vi "Handle Messages.vi"(8 "error in (no error)":errorcluster, 9 "Message Data":variant, 10 "Message":string, 11 "Person In":refnum<class "Person.lvclass">) -> (0 "error out":errorcluster, 3 "Person Out":refnum<class "Person.lvclass">)   [LabVIEW 2020, in "Person.lvclass"]
uses:
  Person.lvclass
  C:/Program Files (x86)/National Instruments/LabVIEW 2020/vi.lib/Asteme/Triarc Framework/Process/Process.lvclass
  Person.lvclass/Person.ctl
  <vilib>/Asteme/Triarc Framework/Process/Process.lvclass/Process.ctl
  <vilib>/Asteme/Triarc Framework/Process/Public/Lifecycle/Get Lifecycle State.vi
  <vilib>/Utility/error.llb/Clear Errors.vi
  <vilib>/Utility/error.llb/Error Cluster From Error Code.vi
  <vilib>/Asteme/Triarc Framework/View/View.lvclass
  <vilib>/Asteme/Triarc Framework/Process/Process.lvclass
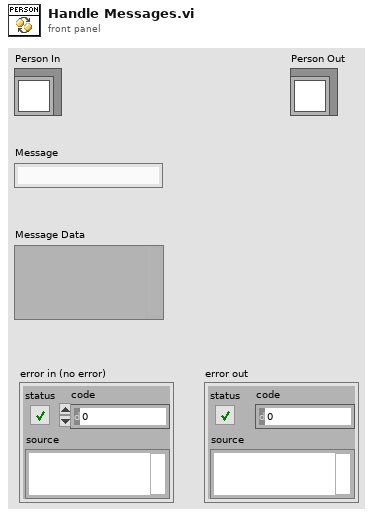
[diagram p1: front panel]
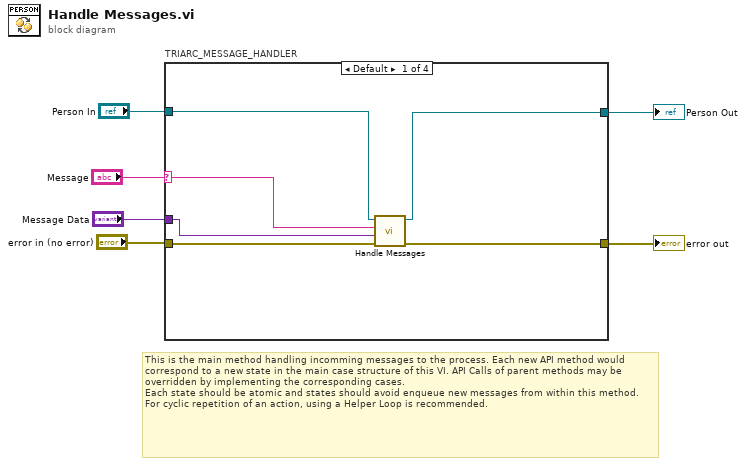
[diagram p0: block diagram]
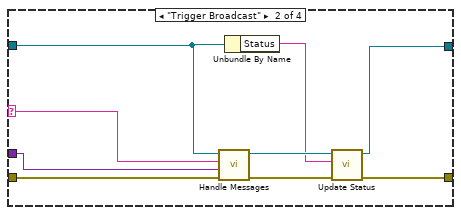
[diagram p2: hidden frame]
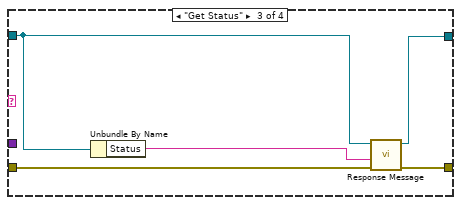
[diagram p3: hidden frame]
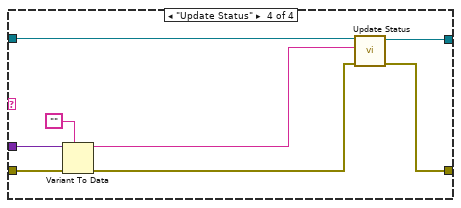
[diagram p4: hidden frame]
diagram:
  # "This is the main method handling incomming messages to the process. Each new API method would correspond to a new state in the main case structure of this VI. API Calls of parent methods may be overridden by implementing the corresponding cases.\nEach state should be atomic and states should avoid enqueue new messages from within this method. For cyclic repetition of an action, using a Helper Loop is recommended."
  n1 = case "TRIARC_MESSAGE_HANDLER" shown="Default" "Message" {
    selector: "Message" -> [w10 w20 _ _]
    tunnel: "error in (no error)" -> [w9 w19 w25 w30]
    tunnel: "Person In" -> [w12 w14 w24 w27]
    tunnel: "Message Data" -> [w11 w21 _ w33]
    tunnel: [w8 w17 w22 w28] -> w2
    tunnel: [w7 w15 w23 w29] -> w1
    frame Default {
      n2 = call-parent "Handle Messages.vi"("error in (no error)"=w9, "Message Data"=w11, "Message"=w10, "View In"=w12) -> ("error out"=w8:errorcluster, "View Out"=w7:refnum<class "Person.lvclass">)  [unwired: 6 in]
    }
    frame "Trigger Broadcast" {
      n3 = call-parent "Handle Messages.vi"("error in (no error)"=w19, "Message Data"=w21, "Message"=w20, "View In"=w14) -> ("error out"=w18:errorcluster, "View Out"=w16:refnum<class "Person.lvclass">)  [unwired: 6 in]
      n4 = Unbundle By Name(w14) -> ("Status"=w13:string)
      n5 = call "Update Status.vi"("error in (no error)"=w18, "Status"=w13, "Person In"=w16) -> ("error out"=w17:errorcluster, "Person Out"=w15:refnum<class "Person.lvclass">)  [unwired: 7 in]
    }
    frame "Get Status" {
      n6 = Unbundle By Name(w24) -> ("Status"=w26:string)
      n7 = call <vilib>:"Response Message.vi"("error in (no error)"=w25, "Response Message Data"=w26, "Process In"=w24) -> ("error out"=w22:errorcluster, "Process Out"=w23:refnum<class "Person.lvclass">)  [unwired: 7 in]
    }
    frame "Update Status" {
      n8 = Variant To Data(error in=w30, type="", Variant=w33) -> (data=w31:string, error out=w34:errorcluster)
      n9 = call "Update Status.vi"("error in (no error)"=w34, "Status"=w31, "Person In"=w27) -> ("error out"=w28:errorcluster, "Person Out"=w29:refnum<class "Person.lvclass">)  [unwired: 7 in]
    }
  }
  "error out" <- w2
  "Person Out" <- w1
